vi "F510-D.vi"(8 "error in (no error)":errorcluster, 10 "Deadzone Scale Cluster":cluster{"Scale":dbl, "Deadzone":dbl}={"Scale"=1.0, "Deadzone"=0.1}, 11 "refnum name":string) -> (0 "error out":errorcluster, 1 "D-Pad Buttons":T1, 2 "Right Stick":cluster{"X":dbl, "Y":dbl}, 3 "Left Stick":cluster{"X":dbl, "Y":dbl}, 4 "Buttons":T2)   [LabVIEW 2014]
uses:
  <vilib>/Rock Robotics/WPI/Joystick/WPI_JoystickGetSetRefNum.vi
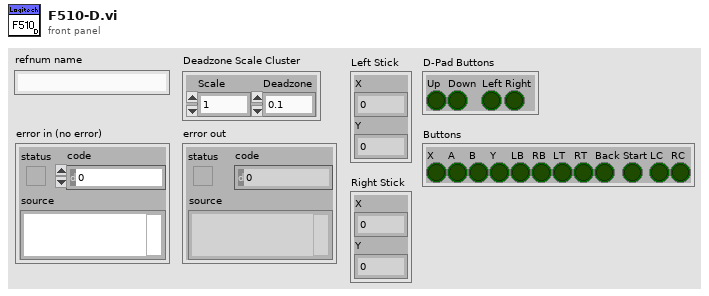
[diagram p1: front panel]
types:
  T1 = cluster{"Up":bool, "Down":bool, "Left":bool, "Right":bool}
  T2 = cluster{"X":bool, "A":bool, "B":bool, "Y":bool, "LB":bool, "RB":bool, "LT":bool, "RT":bool, "Back":bool, "Start":bool, "LC":bool, "RC":bool}
  T3 = typedef "WPI_JoystickDevRef.ctl" = cluster{"Device":T4}
  T4 = typedef "WPI_JoystickDeviceEnum.ctl" = enum16{"USB 0", "USB 1", "USB 2", "USB 3", "USB 4", "USB 5"}
  T5 = cluster{"Up":bool, "Down":bool, "Left":bool, "Right":bool}[]
  T6 = cluster{"Buttons[0]":bool, "Buttons[1]":bool, "Buttons[2]":bool, "Buttons[3]":bool, "Buttons[4]":bool, "Buttons[5]":bool, "Buttons[6]":bool, "Buttons[7]":bool, "Buttons[8]":bool, "Buttons[9]":bool, "Buttons[10]":bool, "Buttons[11]":bool}
  T7 = cluster{"[0]":dbl, "[1]":dbl, "[2]":dbl, "[3]":dbl}
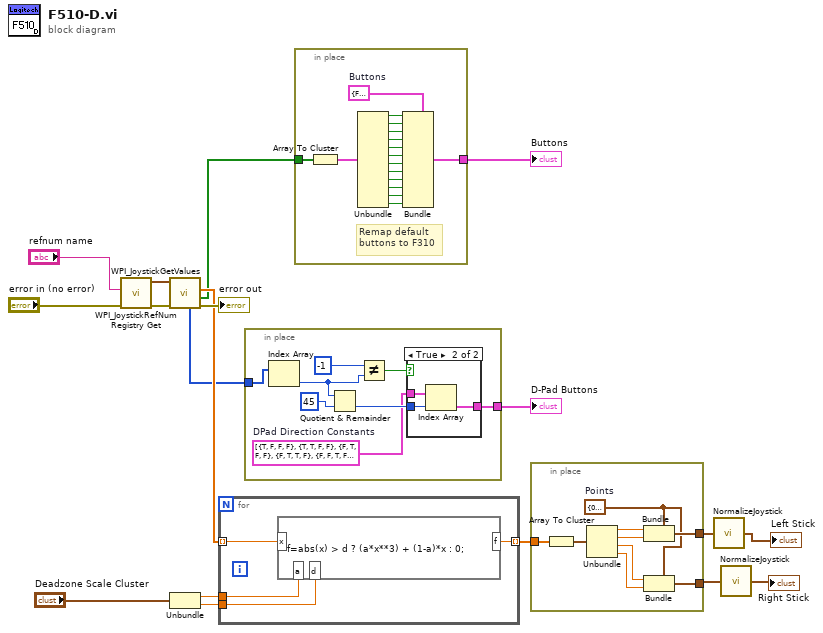
[diagram p0: block diagram]
diagram:
  n1 = call <vilib>:"WPI_JoystickRefNum Registry Get.vi"("error in (no error)"="error in (no error)", "refnum name"="refnum name") -> ("error out"=w15:errorcluster, "JoystickDevRef"=w16:T3)  [unwired: 8 in]
  n2 = call <vilib>:"WPI_JoystickGetValues.vi"("error in (no error)"=w15, "JoystickDevRef"=w16) -> ("error out"=→"error out":errorcluster, "Buttons"=w7:bool[], "Axes"=w13:dbl[], "POVs"=w6:i16[])  [unwired: 5 in, 1 out]
  n3 = Unbundle("Deadzone Scale Cluster") -> ("Scale"=w11:dbl, "Deadzone"=w10:dbl)
  n4 = for {
    tunnel: w13 -> [w22] mode=indexing
    tunnel: w11 -> [w21]
    tunnel: w10 -> [w20]
    tunnel: [w19] -> w9 mode=indexing
    n5 = formula code="f=abs(x) > d ? (a*x**3) + (1-a)*x : 0;"("x"=w22, "d"=w20, "a"=w21) -> ("f"=w19:dbl)
  }
  n6 = in-place {
    in-place-border: w6 -> [w30]
    in-place-border: [w25] -> w5
    w26 = T5 [{"Up"=TRUE, "Down"=FALSE, "Left"=FALSE, "Right"=FALSE}, {"Up"=TRUE, "Down"=TRUE, "Left"=FALSE, "Right"=FALSE}, {"Up"=FALSE, "Down"=TRUE, "Left"=FALSE, "Right"=FALSE}, {"Up"=FALSE, "Down"=TRUE, "Left"=TRUE, "Right"=FALSE}, {"Up"=FALSE, "Down"=FALSE, "Left"=TRUE, "Right"=FALSE}, {"Up"=FALSE, "Down"=FALSE, "Left"=TRUE, "Right"=TRUE}, {"Up"=FALSE, "Down"=FALSE, "Left"=FALSE, "Right"=TRUE}, {"Up"=TRUE, "Down"=FALSE, "Left"=FALSE, "Right"=TRUE}]  # DPad Direction Constants
    n7 = Index Array(array=w30) -> (element=w24:i16)  [unwired: 1 in]
    n8 = Quotient & Remainder(x=w24, y=u16 45) -> (floor(x/y)=w28:u16)  [unwired: 1 out]
    n9 = Not Equal?(x=i16 -1, y=w24) -> (x != y?=w27:bool)
    n10 = case shown="True" w27 {
      tunnel: w28 -> [_ w33]
      tunnel: w26 -> [_ w32]
      tunnel: [_ w31] -> w25
      frame False {
      }
      frame True {
        n11 = Index Array(array=w32, index=w33) -> (element=w31:T1)
      }
    }
  }
  "D-Pad Buttons" <- w5
  n12 = in-place {
    in-place-border: w7 -> [w34]
    in-place-border: [w36] -> w8
    w49 = T2 {"X"=FALSE, "A"=FALSE, "B"=FALSE, "Y"=FALSE, "LB"=FALSE, "RB"=FALSE, "LT"=FALSE, "RT"=FALSE, "Back"=FALSE, "Start"=FALSE, "LC"=FALSE, "RC"=FALSE}  # Buttons
    # "Remap default\nbuttons to F310"
    n13 = Array To Cluster(array=w34) -> (cluster=w35:T6)
    n14 = Unbundle(w35) -> ("Buttons[0]"=w48:bool, "Buttons[1]"=w47:bool, "Buttons[2]"=w46:bool, "Buttons[3]"=w45:bool, "Buttons[4]"=w44:bool, "Buttons[5]"=w43:bool, "Buttons[6]"=w42:bool, "Buttons[7]"=w41:bool, "Buttons[8]"=w40:bool, "Buttons[9]"=w39:bool, "Buttons[10]"=w38:bool, "Buttons[11]"=w37:bool)
    n15 = Bundle(cluster=w49, "X"=w48, "A"=w47, "B"=w46, "Y"=w45, "LB"=w44, "RB"=w43, "LT"=w42, "RT"=w41, "Back"=w40, "Start"=w39, "LC"=w38, "RC"=w37) -> (w36:T2)
  }
  "Buttons" <- w8
  n16 = in-place {
    in-place-border: w9 -> [w53]
    in-place-border: [w52] -> w2
    in-place-border: [w51] -> w4
    w50 = cluster{"X":dbl, "Y":dbl} {"X"=0.0, "Y"=0.0}  # Points
    n17 = Array To Cluster(array=w53) -> (cluster=w58:T7)
    n18 = Unbundle(w58) -> ("[0]"=w54:dbl, "[1]"=w55:dbl, "[2]"=w56:dbl, "[3]"=w57:dbl)
    n19 = Bundle(cluster=w50, "X"=w54, "Y"=w55) -> (w51:cluster{"X":dbl, "Y":dbl})
    n20 = Bundle(cluster=w50, "X"=w56, "Y"=w57) -> (w52:cluster{"X":dbl, "Y":dbl})
  }
  n21 = call "NormalizeJoystick.vi"("joystick"=w4) -> ("normalized joystick"=→"Left Stick":cluster{"x":dbl, "y":dbl})
  n22 = call "NormalizeJoystick.vi"("joystick"=w2) -> ("normalized joystick"=→"Right Stick":cluster{"x":dbl, "y":dbl})
